vi "WD_ReveiveName.vi"() -> (3 "ArrayOut":string[](array[string]))   [LabVIEW 2011]
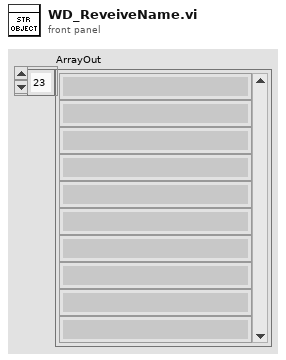
[diagram p1: front panel]
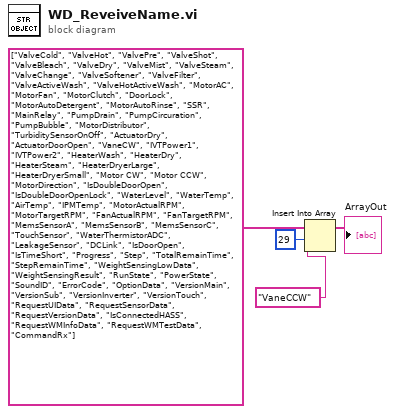
[diagram p0: block diagram]
diagram:
  n1 = Insert Into Array(array=string[] ["ValveCold", "ValveHot", "ValvePre", "ValveShot", "ValveBleach", "ValveDry", "ValveMist", "ValveSteam", "ValveChange", "ValveSoftener", "ValveFilter", "ValveActiveWash", "ValveHotActiveWash", "MotorAC", "MotorFan", "MotorClutch", "DoorLock", "MotorAutoDetergent", "MotorAutoRinse", "SSR", "MainRelay", "PumpDrain", "PumpCircuration", "PumpBubble", "MotorDistributor", "TurbiditySensorOnOff", "ActuatorDry", "ActuatorDoorOpen", "VaneCW", "IVTPower1", "IVTPower2", "HeaterWash", "HeaterDry", "HeaterSteam", "HeaterDryerLarge", "HeaterDryerSmall", "Motor CW", "Motor CCW", "MotorDirection", "IsDoubleDoorOpen", "IsDoubleDoorOpenLock", "WaterLevel", "WaterTemp", "AirTemp", "IPMTemp", "MotorActualRPM", "MotorTargetRPM", "FanActualRPM", "FanTargetRPM", "MemsSensorA", "MemsSensorB", "MemsSensorC", "TouchSensor", "WaterThermistorADC", "LeakageSensor", "DCLink", "IsDoorOpen", "IsTimeShort", "Progress", "Step", "TotalRemainTime", "StepRemainTime", "WeightSensingLowData", "WeightSensingResult", "RunState", "PowerState", "SoundID", "ErrorCode", "OptionData", "VersionMain", "VersionSub", "VersionInverter", "VersionTouch", "RequestUIData", "RequestSensorData", "RequestVersionData", "IsConnectedHASS", "RequestWMInfoData", "RequestWMTestData", "CommandRx"], index=29 ("索引"), new element="VaneCCW") -> (→"ArrayOut":string[])
